vi "Read_CSV_Dataset.vi"(8 "error in (no error)":errorcluster, 11 "CSV Folder Path":path) -> (0 "error out":errorcluster, 3 "Labels Map":map{string, sgl[]}(c390))   [LabVIEW 2020]
uses:
  <vilib>/Utility/file.llb/Read Delimited Spreadsheet (string).vi
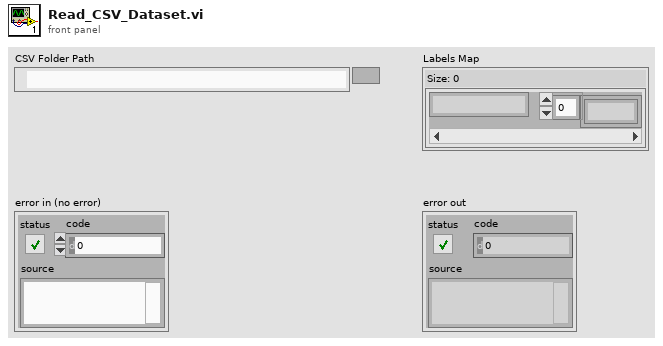
[diagram p1: front panel]
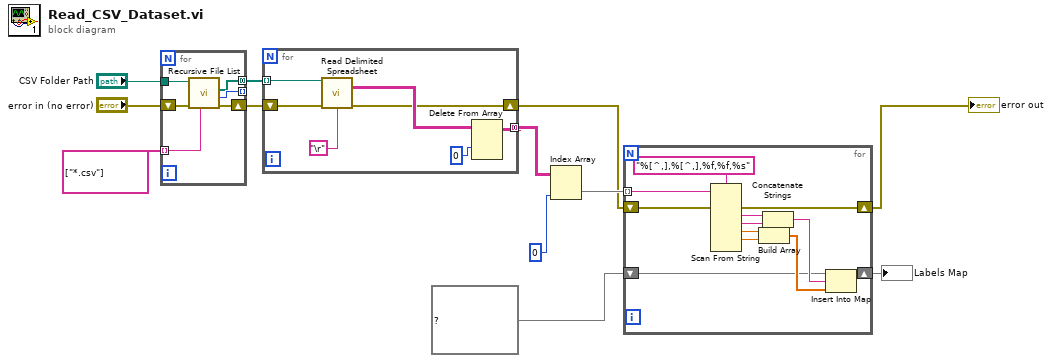
[diagram p0: block diagram]
diagram:
  n1 = for {
    tunnel: string[] ["*.csv"] ("pattern") -> [w18] mode=indexing
    tunnel: "CSV Folder Path" -> [w16]
    tunnel: [w15] -> _ mode=indexing
    tunnel: [w14] -> w12 mode=concatenating
    shift-right: [w13] -> w3
    shift-left: "error in (no error)" -> [w17]
    n2 = call <vilib>:"Recursive File List.vi"("pattern"=w18, "error in (no error)"=w17, "Folder Path"=w16) -> ("error out"=w13:errorcluster, "Number of Files"=w15:i32, "All Files in Dir"=w14:path[])  [unwired: 4 in, 2 out]
  }
  n3 = for {
    tunnel: w12 -> [w25] mode=indexing
    tunnel: [w22] -> w10 mode=concatenating
    shift-right: [w19] -> w2
    shift-left: w3 -> [w20]
    n4 = call-poly <vilib>:"Read Delimited Spreadsheet.vi"("file path (dialog if empty)"=w25, "error in (no error)"=w20, "delimiter (\\t)"="\r") -> ("all rows"=w23:string[][], "error out"=w19:errorcluster)  [unwired: 7 in, 4 out]
    n5 = Delete From Array(array=w23, index (row)=0 ("disabled index (col)")) -> (array with subset deleted=w22:string[][])  [unwired: 2 in, 1 out]
  }
  n6 = Index Array(array=w10, index (col)=0 ("disabled index (col)")) -> (element=w9:string[])  [unwired: 1 in]
  n7 = for {
    tunnel: w9 -> [w37] mode=indexing
    shift-right: [w30] -> w4
    shift-left: map{string, sgl[]} {} ("map") -> [w31]
    shift-right: [w26] -> w1
    shift-left: w2 -> [w27]
    n8 = Scan From String(format string="%[^,],%[^,],%f,%f,%s", input string=w37, error in=w27) -> (error out=w26:errorcluster, output 1=w36:string, output 2=w28:string, output 3=w35:dbl, output 4=w34:dbl)  [unwired: 7 in, 2 out]
    n9 = Build Array(w35, w34) -> (w32:dbl[])
    n10 = Concatenate Strings(w36, w28) -> (w33:string)
    n11 = Insert Into Map(map in=w31, key=w33, value=w32) -> (map out=w30:map{string, sgl[]})  [unwired: 2 out]
  }
  "Labels Map" <- w4
  "error out" <- w1
